vi "Run_Point_Step.vi"(8 "error in (no error)":errorcluster, 9 "Producer In":T1={"Temps(K)"=[], "Fields(T)"=[], "Sweep States"=enum."1. Idle", "PointStep"=enum."1. Scan_1", "Current Field"=0.0, "Current Temp"=0.0, "Expected_ACK"=enum."1. None", "ACK"=enum."1. None", "AfterAckStep"=enum."1. Idle", "Current Index Field"=0, "Current Index Temp"=0, "ACK Structure "=enum."Inner"}, 10 "ScanQ In":refnum<queue>, 11 "SweepQ In":refnum<queue>) -> (0 "error out":errorcluster, 1 "Producer Out":T1={"Temps(K)"=[], "Fields(T)"=[], "Sweep States"=enum."1. Idle", "PointStep"=enum."1. Scan_1", "Current Field"=0.0, "Current Temp"=0.0, "Expected_ACK"=enum."1. None", "ACK"=enum."1. None", "AfterAckStep"=enum."1. Idle", "Current Index Field"=0, "Current Index Temp"=0, "ACK Structure "=enum."Inner"}, 2 "ScanQ Out":refnum<queue>, 3 "SweepQ Out":refnum<queue>)   [LabVIEW 2025]
uses:
  CTLS/Sweeper.ctl
  CTLS/Scan_Params (QMH).ctl
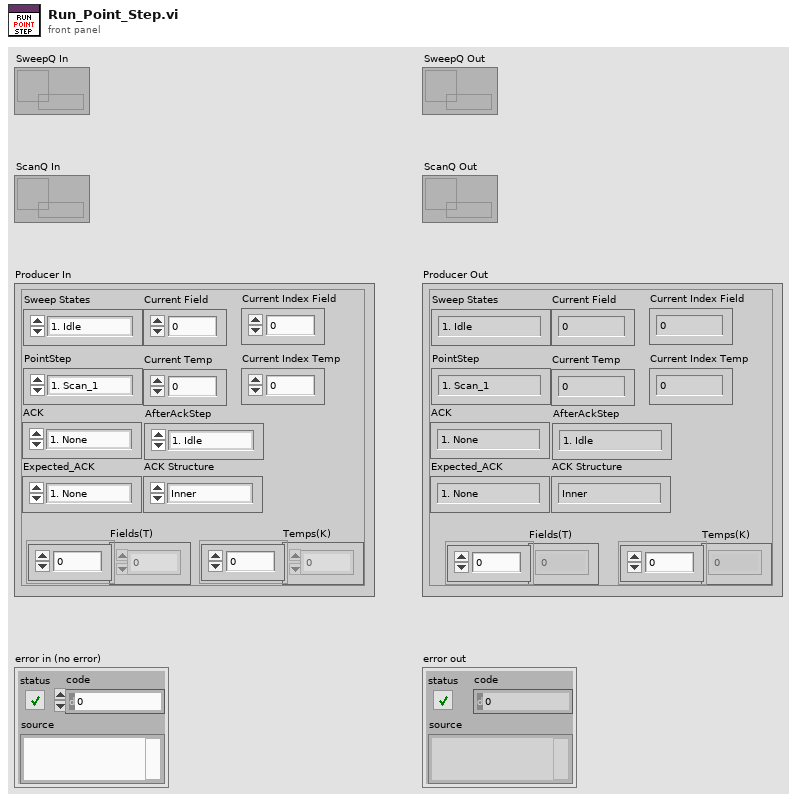
[diagram p1: front panel]
types:
  T1 = typedef "Sweeper.ctl" = cluster{"Temps(K)":dbl[], "Fields(T)":dbl[], "Sweep States":enum16{"1. Idle", "2. Start", "3. Apply_Config", "4. Run_Point_Step", "5. Wait ACK", "6. Next Field", "7. Next Temp", "8. Stop"}, "PointStep":enum16{"1. Init_Bias", "2. Init_Scan", "3. Field_Stable", "4. Temp_stable", "1. Scan_1", "2. DC_SF_1", "3. DC_BS_1", "4. Bias", "5. Scan_2", "6. DC_SF_2", "7. DC_BS_2", "8. Done"}, "Current Field":dbl, "Current Temp":dbl, "Expected_ACK":enum16{"1. None", "2. TempStable", "3. FieldStable", "4. ConfigApplied", "5. ScanDone", "6. BiasDone", "7. DriftDone (SF)", "8. DrifDone (BS)", "9. Done"}, "ACK":enum16{"1. None", "2. TempStable", "3. FieldStable", "4. ConfigApplied", "5. ScanDone", "6. BiasDone", "7. DriftDone (SF)", "8. DrifDone (BS)", "9. Done"}, "AfterAckStep":enum16{"1. Idle", "2. Start", "3. Apply_Config", "4. Run_Point_Step", "5. Wait ACK", "6. Next Field", "7. Next Temp", "8. Stop"}, "Current Index Field":i32, "Current Index Temp":i32, "ACK Structure ":enum16{"Inner", "Outer"}}
  T2 = enum16{"1. Init_Bias", "2. Init_Scan", "3. Field_Stable", "4. Temp_stable", "1. Scan_1", "2. DC_SF_1", "3. DC_BS_1", "4. Bias", "5. Scan_2", "6. DC_SF_2", "7. DC_BS_2", "8. Done"}
  T3 = enum16{"1. Idle", "2. Start", "3. Apply_Config", "4. Run_Point_Step", "5. Wait ACK", "6. Next Field", "7. Next Temp", "8. Stop"}
  T4 = enum16{"1. BIAS", "2. POLL BIAS", "3. SCAN", "4. SCAN_IDLE", "5. Drift_Correct (SF)", "6. Drift_Correct (BS)", "7. STOP"}
  T5 = enum16{"1. None", "2. TempStable", "3. FieldStable", "4. ConfigApplied", "5. ScanDone", "6. BiasDone", "7. DriftDone (SF)", "8. DrifDone (BS)", "9. Done"}
  T6 = typedef "Scan_Params (QMH).ctl" = cluster{"Setpoint (I)":dbl[], "Bias (V)":dbl[], "Number of scans":u8, "Port number (3364)":u32, "Avoid zero threshold (V)":dbl, "Current State":enum16{"1. BIAS", "2. POLL BIAS", "3. SCAN", "4. SCAN_IDLE", "5. Drift_Correct (SF)", "6. Drift_Correct (BS)", "7. STOP"}}
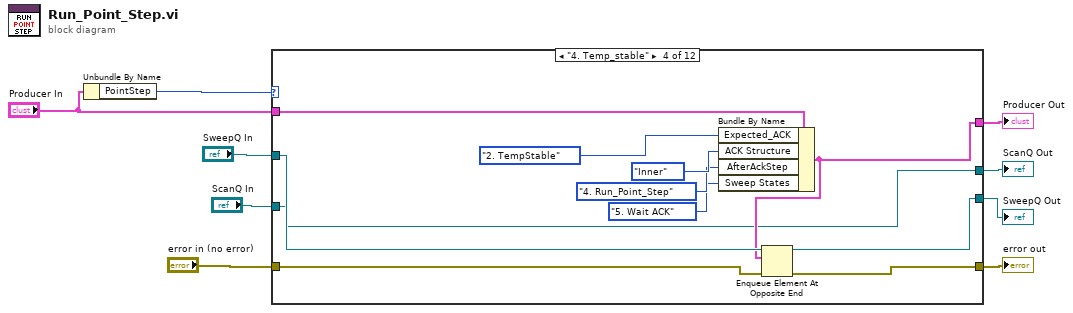
[diagram p0: block diagram]
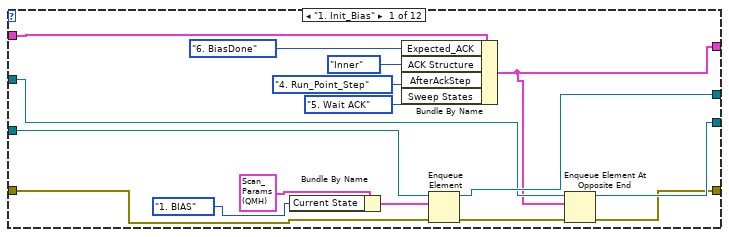
[diagram p2: hidden frame]
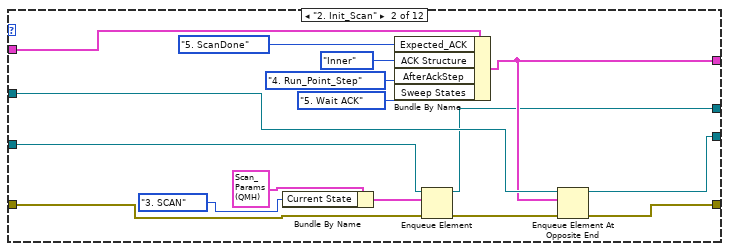
[diagram p3: hidden frame]
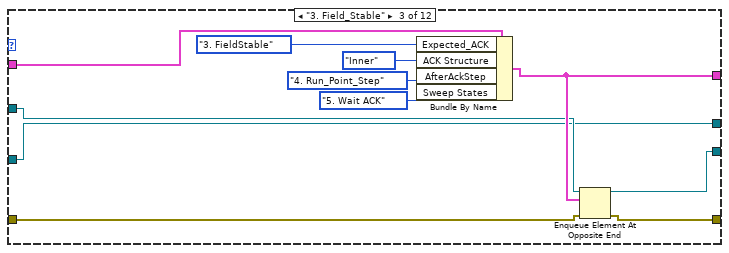
[diagram p4: hidden frame]
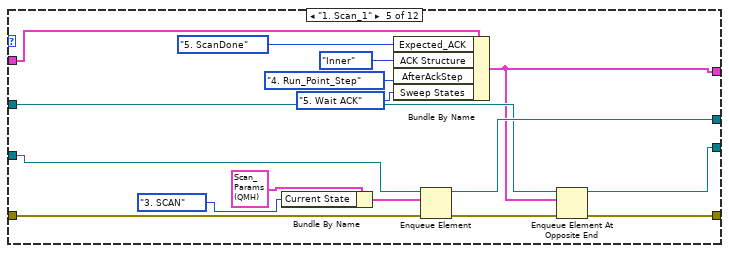
[diagram p5: hidden frame]
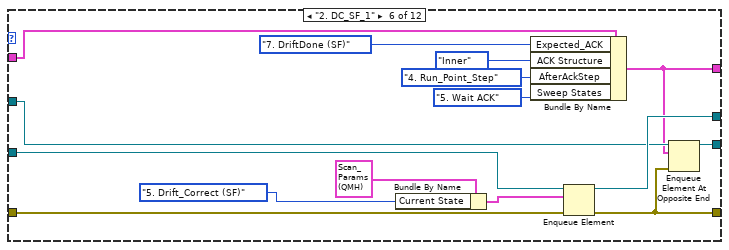
[diagram p6: hidden frame]
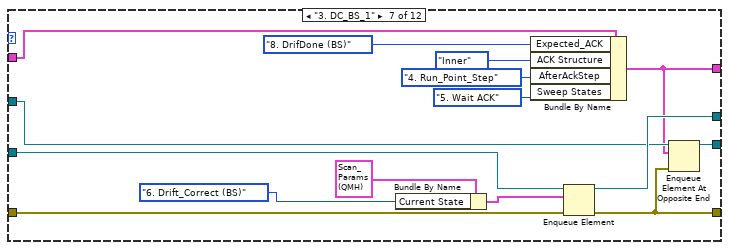
[diagram p7: hidden frame]
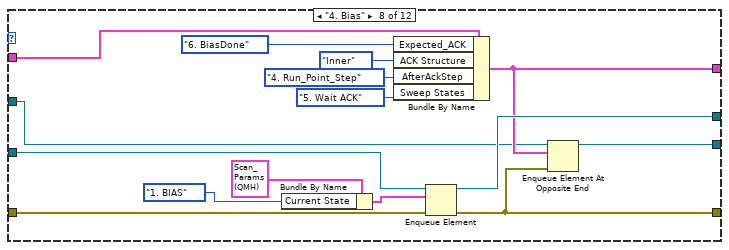
[diagram p8: hidden frame]
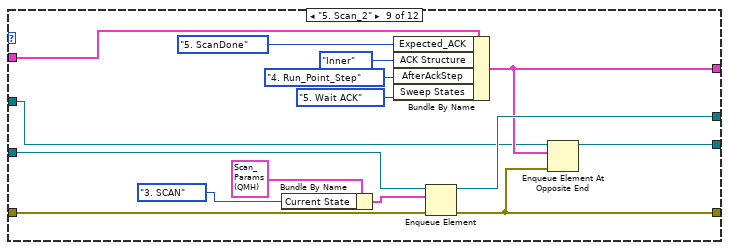
[diagram p9: hidden frame]
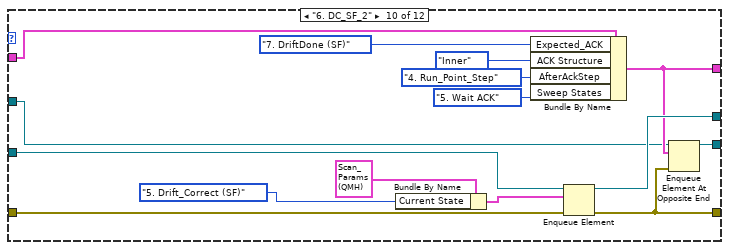
[diagram p10: hidden frame]
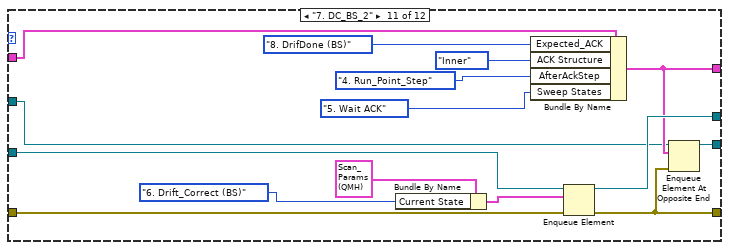
[diagram p11: hidden frame]
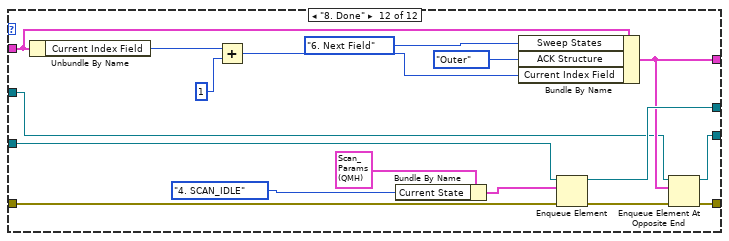
[diagram p12: hidden frame]
diagram:
  n1 = Unbundle By Name("Producer In") -> ("PointStep"=w5:T2)
  n2 = case shown="\"4. Temp_stable\"" w5 {
    tunnel: "ScanQ In" -> [w14 w27 w43 w53 w79 w88 w102 w118 w133 w148 w163 w181]
    tunnel: "Producer In" -> [w17 w33 w48 w59 w76 w85 w104 w119 w131 w149 w164 w174]
    tunnel: [w11 w30 w47 w56 w68 w83 w98 w115 w130 w145 w160 w180] -> w8
    tunnel: "error in (no error)" -> [w10 w26 w42 w54 w73 w89 w101 w117 w132 w147 w162 w182]
    tunnel: [w16 w28 w43 w53 w72 w90 w103 w116 w134 w146 w161 w183] -> w4
    tunnel: [w15 w32 w45 w57 w70 w86 w100 w113 w128 w143 w159 w178] -> w3
    tunnel: "SweepQ In" -> [w13 w31 w46 w58 w69 w84 w99 w114 w129 w144 w158 w179]
    tunnel: [w12 w29 w44 w55 w66 w82 w97 w112 w127 w142 w157 w176] -> w1
    frame "1. Init_Bias" {
      n3 = Bundle By Name(cluster=T6 {"Setpoint (I)"=[], "Bias (V)"=[], "Number of scans"=1, "Port number (3364)"=3364, "Avoid zero threshold (V)"=0.004999999888241291, "Current State"=enum."1. BIAS"} ("Scan Parameters"), "Current State"=T4."1. BIAS") -> (w24:T6)
      n4 = Bundle By Name(cluster=w17, "Expected_ACK"=T5."6. BiasDone", "ACK Structure"=enum16{"Inner", "Outer"}."Inner", "AfterAckStep"=T3."4. Run_Point_Step", "Sweep States"=T3."5. Wait ACK") -> (w11:T1)
      n5 = Enqueue Element(queue=w14, element=w24, error in (no error)=w10) -> (queue out=w16:refnum<queue>, error out=w20:errorcluster)  [unwired: 1 in, 1 out]
      n6 = Enqueue Element At Opposite End(queue=w13, element=w11, error in (no error)=w20) -> (queue out=w15:refnum<queue>, error out=w12:errorcluster)  [unwired: 1 in, 1 out]
    }
    frame "2. Init_Scan" {
      n7 = Bundle By Name(cluster=T6 {"Setpoint (I)"=[], "Bias (V)"=[], "Number of scans"=1, "Port number (3364)"=3364, "Avoid zero threshold (V)"=0.004999999888241291, "Current State"=enum."1. BIAS"} ("Scan Parameters"), "Current State"=T4."3. SCAN") -> (w40:T6)
      n8 = Bundle By Name(cluster=w33, "Expected_ACK"=T5."5. ScanDone", "ACK Structure"=enum16{"Inner", "Outer"}."Inner", "AfterAckStep"=T3."4. Run_Point_Step", "Sweep States"=T3."5. Wait ACK") -> (w30:T1)
      n9 = Enqueue Element(queue=w27, element=w40, error in (no error)=w26) -> (queue out=w28:refnum<queue>, error out=w36:errorcluster)  [unwired: 1 in, 1 out]
      n10 = Enqueue Element At Opposite End(queue=w31, element=w30, error in (no error)=w36) -> (queue out=w32:refnum<queue>, error out=w29:errorcluster)  [unwired: 1 in, 1 out]
    }
    frame "3. Field_Stable" {
      n11 = Bundle By Name(cluster=w48, "Expected_ACK"=T5."3. FieldStable", "ACK Structure"=enum16{"Inner", "Outer"}."Inner", "AfterAckStep"=T3."4. Run_Point_Step", "Sweep States"=T3."5. Wait ACK") -> (w47:T1)
      n12 = Enqueue Element At Opposite End(queue=w46, element=w47, error in (no error)=w42) -> (queue out=w45:refnum<queue>, error out=w44:errorcluster)  [unwired: 1 in, 1 out]
    }
    frame "4. Temp_stable" {
      n13 = Bundle By Name(cluster=w59, "Expected_ACK"=T5."2. TempStable", "ACK Structure"=enum16{"Inner", "Outer"}."Inner", "AfterAckStep"=T3."4. Run_Point_Step", "Sweep States"=T3."5. Wait ACK") -> (w56:T1)
      n14 = Enqueue Element At Opposite End(queue=w58, element=w56, error in (no error)=w54) -> (queue out=w57:refnum<queue>, error out=w55:errorcluster)  [unwired: 1 in, 1 out]
    }
    frame "1. Scan_1" {
      n15 = Bundle By Name(cluster=T6 {"Setpoint (I)"=[], "Bias (V)"=[], "Number of scans"=1, "Port number (3364)"=3364, "Avoid zero threshold (V)"=0.004999999888241291, "Current State"=enum."1. BIAS"} ("Scan Parameters"), "Current State"=T4."3. SCAN") -> (w77:T6)
      n16 = Bundle By Name(cluster=w76, "Expected_ACK"=T5."5. ScanDone", "ACK Structure"=enum16{"Inner", "Outer"}."Inner", "AfterAckStep"=T3."4. Run_Point_Step", "Sweep States"=T3."5. Wait ACK") -> (w68:T1)
      n17 = Enqueue Element(queue=w79, element=w77, error in (no error)=w73) -> (queue out=w72:refnum<queue>, error out=w67:errorcluster)  [unwired: 1 in, 1 out]
      n18 = Enqueue Element At Opposite End(queue=w69, element=w68, error in (no error)=w67) -> (queue out=w70:refnum<queue>, error out=w66:errorcluster)  [unwired: 1 in, 1 out]
    }
    frame "2. DC_SF_1" {
      n19 = Bundle By Name(cluster=T6 {"Setpoint (I)"=[], "Bias (V)"=[], "Number of scans"=1, "Port number (3364)"=3364, "Avoid zero threshold (V)"=0.004999999888241291, "Current State"=enum."1. BIAS"} ("Scan Parameters"), "Current State"=T4."5. Drift_Correct (SF)") -> (w93:T6)
      n20 = Bundle By Name(cluster=w85, "Expected_ACK"=T5."7. DriftDone (SF)", "ACK Structure"=enum16{"Inner", "Outer"}."Inner", "AfterAckStep"=T3."4. Run_Point_Step", "Sweep States"=T3."5. Wait ACK") -> (w83:T1)
      n21 = Enqueue Element(queue=w88, element=w93, error in (no error)=w89) -> (queue out=w90:refnum<queue>, error out=w82:errorcluster)  [unwired: 1 in, 1 out]
      n22 = Enqueue Element At Opposite End(queue=w84, element=w83, error in (no error)=w82) -> (queue out=w86:refnum<queue>)  [unwired: 1 in, 2 out]
    }
    frame "3. DC_BS_1" {
      n23 = Bundle By Name(cluster=T6 {"Setpoint (I)"=[], "Bias (V)"=[], "Number of scans"=1, "Port number (3364)"=3364, "Avoid zero threshold (V)"=0.004999999888241291, "Current State"=enum."1. BIAS"} ("Scan Parameters"), "Current State"=T4."6. Drift_Correct (BS)") -> (w108:T6)
      n24 = Bundle By Name(cluster=w104, "Expected_ACK"=T5."8. DrifDone (BS)", "ACK Structure"=enum16{"Inner", "Outer"}."Inner", "AfterAckStep"=T3."4. Run_Point_Step", "Sweep States"=T3."5. Wait ACK") -> (w98:T1)
      n25 = Enqueue Element(queue=w102, element=w108, error in (no error)=w101) -> (queue out=w103:refnum<queue>, error out=w97:errorcluster)  [unwired: 1 in, 1 out]
      n26 = Enqueue Element At Opposite End(queue=w99, element=w98, error in (no error)=w97) -> (queue out=w100:refnum<queue>)  [unwired: 1 in, 2 out]
    }
    frame "4. Bias" {
      n27 = Bundle By Name(cluster=T6 {"Setpoint (I)"=[], "Bias (V)"=[], "Number of scans"=1, "Port number (3364)"=3364, "Avoid zero threshold (V)"=0.004999999888241291, "Current State"=enum."1. BIAS"} ("Scan Parameters"), "Current State"=T4."1. BIAS") -> (w123:T6)
      n28 = Bundle By Name(cluster=w119, "Expected_ACK"=T5."6. BiasDone", "ACK Structure"=enum16{"Inner", "Outer"}."Inner", "AfterAckStep"=T3."4. Run_Point_Step", "Sweep States"=T3."5. Wait ACK") -> (w115:T1)
      n29 = Enqueue Element(queue=w118, element=w123, error in (no error)=w117) -> (queue out=w116:refnum<queue>, error out=w112:errorcluster)  [unwired: 1 in, 1 out]
      n30 = Enqueue Element At Opposite End(queue=w114, element=w115, error in (no error)=w112) -> (queue out=w113:refnum<queue>)  [unwired: 1 in, 2 out]
    }
    frame "5. Scan_2" {
      n31 = Bundle By Name(cluster=T6 {"Setpoint (I)"=[], "Bias (V)"=[], "Number of scans"=1, "Port number (3364)"=3364, "Avoid zero threshold (V)"=0.004999999888241291, "Current State"=enum."1. BIAS"} ("Scan Parameters"), "Current State"=T4."3. SCAN") -> (w138:T6)
      n32 = Bundle By Name(cluster=w131, "Expected_ACK"=T5."5. ScanDone", "ACK Structure"=enum16{"Inner", "Outer"}."Inner", "AfterAckStep"=T3."4. Run_Point_Step", "Sweep States"=T3."5. Wait ACK") -> (w130:T1)
      n33 = Enqueue Element(queue=w133, element=w138, error in (no error)=w132) -> (queue out=w134:refnum<queue>, error out=w127:errorcluster)  [unwired: 1 in, 1 out]
      n34 = Enqueue Element At Opposite End(queue=w129, element=w130, error in (no error)=w127) -> (queue out=w128:refnum<queue>)  [unwired: 1 in, 2 out]
    }
    frame "6. DC_SF_2" {
      n35 = Bundle By Name(cluster=T6 {"Setpoint (I)"=[], "Bias (V)"=[], "Number of scans"=1, "Port number (3364)"=3364, "Avoid zero threshold (V)"=0.004999999888241291, "Current State"=enum."1. BIAS"} ("Scan Parameters"), "Current State"=T4."5. Drift_Correct (SF)") -> (w153:T6)
      n36 = Bundle By Name(cluster=w149, "Expected_ACK"=T5."7. DriftDone (SF)", "ACK Structure"=enum16{"Inner", "Outer"}."Inner", "AfterAckStep"=T3."4. Run_Point_Step", "Sweep States"=T3."5. Wait ACK") -> (w145:T1)
      n37 = Enqueue Element(queue=w148, element=w153, error in (no error)=w147) -> (queue out=w146:refnum<queue>, error out=w142:errorcluster)  [unwired: 1 in, 1 out]
      n38 = Enqueue Element At Opposite End(queue=w144, element=w145, error in (no error)=w142) -> (queue out=w143:refnum<queue>)  [unwired: 1 in, 2 out]
    }
    frame "7. DC_BS_2" {
      n39 = Bundle By Name(cluster=T6 {"Setpoint (I)"=[], "Bias (V)"=[], "Number of scans"=1, "Port number (3364)"=3364, "Avoid zero threshold (V)"=0.004999999888241291, "Current State"=enum."1. BIAS"} ("Scan Parameters"), "Current State"=T4."6. Drift_Correct (BS)") -> (w168:T6)
      n40 = Bundle By Name(cluster=w164, "Expected_ACK"=T5."8. DrifDone (BS)", "ACK Structure"=enum16{"Inner", "Outer"}."Inner", "AfterAckStep"=T3."4. Run_Point_Step" ("Sweep States"), "Sweep States"=T3."5. Wait ACK" ("AfterAckStep")) -> (w160:T1)
      n41 = Enqueue Element(queue=w163, element=w168, error in (no error)=w162) -> (queue out=w161:refnum<queue>, error out=w157:errorcluster)  [unwired: 1 in, 1 out]
      n42 = Enqueue Element At Opposite End(queue=w158, element=w160, error in (no error)=w157) -> (queue out=w159:refnum<queue>)  [unwired: 1 in, 2 out]
    }
    frame "8. Done" {
      n43 = Unbundle By Name(w174) -> ("Current Index Field"=w170:i32)
      n44 = Add(x=w170, y=1) -> (x+y=w173:i32)
      n45 = Bundle By Name(cluster=T6 {"Setpoint (I)"=[], "Bias (V)"=[], "Number of scans"=1, "Port number (3364)"=3364, "Avoid zero threshold (V)"=0.004999999888241291, "Current State"=enum."1. BIAS"} ("Scan Parameters"), "Current State"=T4."4. SCAN_IDLE") -> (w185:T6)
      n46 = Bundle By Name(cluster=w174, "Sweep States"=T3."6. Next Field", "ACK Structure"=enum16{"Inner", "Outer"}."Outer", "Current Index Field"=w173) -> (w180:T1)
      n47 = Enqueue Element(queue=w181, element=w185, error in (no error)=w182) -> (queue out=w183:refnum<queue>, error out=w177:errorcluster)  [unwired: 1 in, 1 out]
      n48 = Enqueue Element At Opposite End(queue=w179, element=w180, error in (no error)=w177) -> (queue out=w178:refnum<queue>, error out=w176:errorcluster)  [unwired: 1 in, 1 out]
    }
  }
  "error out" <- w1
  "Producer Out" <- w8
  "ScanQ Out" <- w4
  "SweepQ Out" <- w3
